vi "niRFUtil MT UTIL Validate Complex Waveform.vi"(8 "error in (no error)":errorcluster, 11 "Waveform In":T1={"x0"=0.0, "dx"=1.0, "y"=[]} caption="input complex waveform" {"y" format="%.2f"; "dx" format="%^.2e"; "x0" format="%^.2e"}) -> (0 "error out":errorcluster, 1 "error?":bool, 3 "Waveform Out":T1 caption="output complex waveform" {"y" format="%.2f"; "dx" format="%^.2e"; "x0" format="%^.2e"})   [LabVIEW 2015, in "niRFUtil.lvlib"]
doc: "Verifies that the provided Input Complex Waveform is valid based on:\n1. \"dt\" parameter is greater than zero.\n2. Waveform contains values."
uses:
  niRFUtil.lvlib
  Includes/niRFUtil INC Complex Waveform.ctl
  Includes/niRFUtil INC Complex Array.ctl
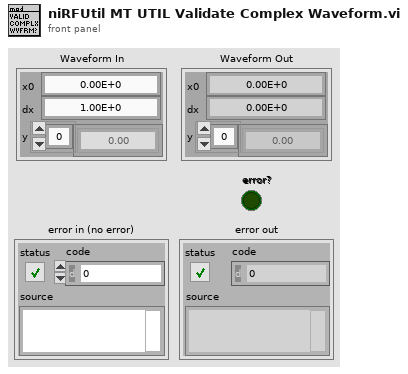
[diagram p1: front panel]
types:
  T1 = typedef "niRFUtil.lvlib/niRFUtil INC Complex Waveform.ctl" = cluster{"x0":dbl, "dx":dbl, "y":T2}
  T2 = typedef "niRFUtil.lvlib/niRFUtil INC Complex Array.ctl" = csg[]
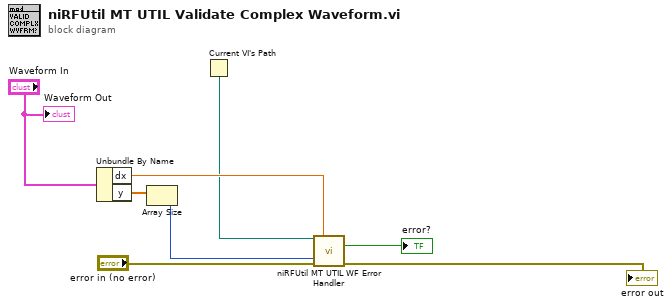
[diagram p0: block diagram]
diagram:
  n1 = Unbundle By Name("Waveform In") -> ("dx"=w3:dbl, "y"=w7:T2)
  n2 = Array Size(array=w7) -> (size(s)=w4:i32)
  n3 = Current VI's Path() -> (path=w2:path)
  n4 = call "niRFUtil MT UTIL WF Error Handler.vi"("path to calling VI"=w2, "dt"=w3, "waveform length (samples)"=w4, "error in (no error)"="error in (no error)") -> ("error?"=→"error?":bool, "error out"=→"error out":errorcluster)  [unwired: 10 out]
  "Waveform Out" <- "Waveform In"
